vi "Get Data.vi"(8 "error in":errorcluster, 11 "Cfg Dev in":refnum<class "CnPt.lvclass">) -> (0 "error out":errorcluster, 2 "Data":refnum<class "Data.lvclass">, 3 "Cfg Dev out":refnum<class "CnPt.lvclass">)   [LabVIEW 2015, in "CnPt.lvclass"]
uses:
  CnPt.lvclass
  <vilib>/MSR Consulting, LLC/General Reuse/Data/Data.lvclass
  <vilib>/MSR Consulting, LLC/General Reuse/Session APIs/Serial/Serial Session.lvclass
  <vilib>/MSR Consulting, LLC/General Reuse/Data/Double/Double.lvclass
  CnPt.lvclass/CnPt.ctl
  <vilib>/MSR Consulting, LLC/General Reuse/Session APIs/Serial/Public/Asynchronous Write.vi
  <vilib>/MSR Consulting, LLC/General Reuse/Session APIs/Serial/Public/Asynchronous Read.vi
  <vilib>/MSR Consulting, LLC/General Reuse/Data/Write measTime.vi
  <vilib>/MSR Consulting, LLC/General Reuse/Data/Double/Write Data.vi
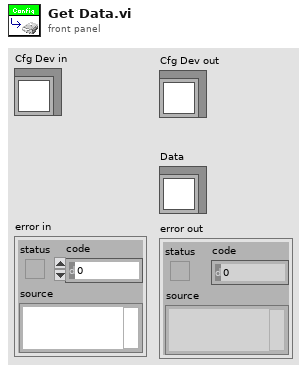
[diagram p1: front panel]
types:
  T1 = typedef "Serial Session.lvclass/Session Handle.ctl" = refnum<data-value>
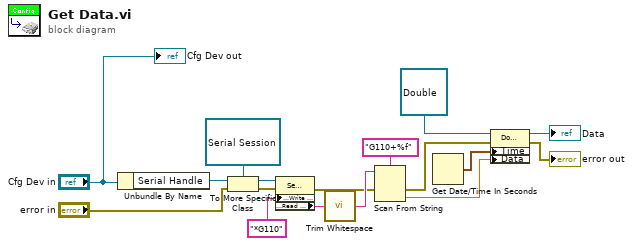
[diagram p0: block diagram]
diagram:
  n1 = Unbundle By Name("Cfg Dev in") -> ("Serial Handle"=w17:T1)
  n2 = To More Specific Class(target class=refnum<data-value> refnum, reference=w17, error in="error in") -> (specific class reference=w15:refnum<data-value>, error out=w13:errorcluster)
  n3 = property class="Serial Session"(reference=w15, error in=w13, "Public:Write - Asynchronous"="*G110" ("format string")) -> (error out=w6:errorcluster, "Public:Read - Asynchronous"=w8:string)  [unwired: 1 out]
  n4 = call <vilib>:"Trim Whitespace.vi"("string"=w8) -> ("trimmed string"=w7:string)  [unwired: 1 in]
  n5 = Scan From String(format string="G110+%f", input string=w7, error in=w6) -> (error out=w5:errorcluster, output 1=w3:dbl)  [unwired: 2 in, 2 out]
  n6 = Get Date/Time In Seconds() -> (seconds since 1Jan1904=w4:timestamp)
  n7 = property class="Double"(reference=refnum<class "Double.lvclass"> refnum ("Base Data Lib:Double"), error in=w5, "Time"=w4, "Data"=w3) -> (reference out=→"Data":refnum<class "Double.lvclass">, error out=→"error out":errorcluster)
  "Cfg Dev out" <- "Cfg Dev in"
